vi "Script Name Wiring.vi"(6 "VI Name":string, 8 "error in":errorcluster, 9 "VI":refnum<vi>, 10 "Terminal Attributes":T1) -> (0 "error out":errorcluster)   [LabVIEW 2025, in "_Rescript.lvlib" / "Msg.lvlib" / "Msg.lvclass"]
uses:
  Msg.lvclass
  Terminal Attributes.ctl
  Attributes.ctl
  <vilib>/Utility/traverseref.llb/TRef TravTarget.ctl
  _Rescript.lvlib
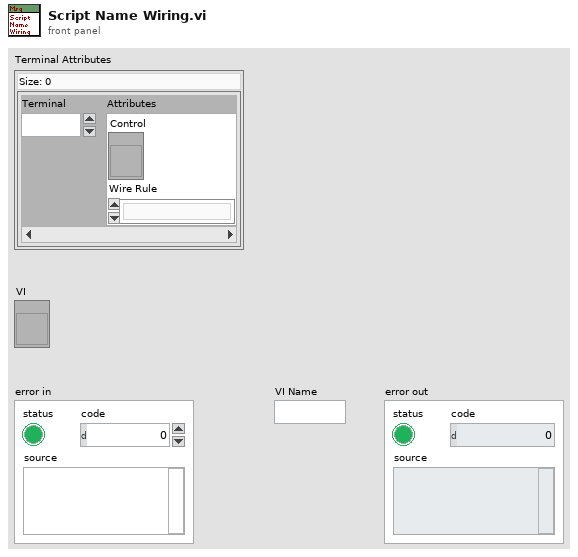
[diagram p1: front panel]
types:
  T1 = typedef "_Rescript.lvlib/Terminal Attributes.ctl" = map{i32, T2}
  T2 = typedef "_Rescript.lvlib/Attributes.ctl" = cluster{"Control":refnum<vi>, "Wire Rule":enum16{"Invalid Wire Rule", "Required", "Recommended", "Optional", "Dynamic Dispatch"}}
  T3 = typedef "TRef TravTarget.ctl" = enum16{"FP", "BD", "Other"}
  T4 = enum16{"Invalid Wire Rule", "Required", "Recommended", "Optional", "Dynamic Dispatch"}
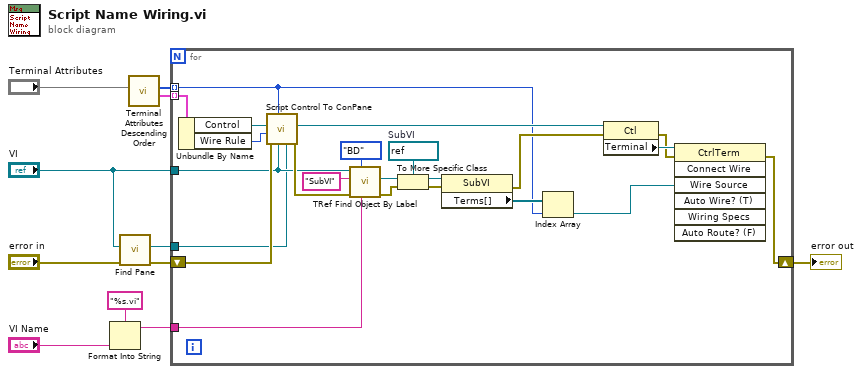
[diagram p0: block diagram]
diagram:
  n1 = Format Into String(format string="%s.vi", "VI Name") -> (resulting string=w4:string)  [unwired: 2 in, 1 out]
  n2 = call "Find Pane.vi"("error in"="error in", "VI Ref"="VI") -> ("error out"=w10:errorcluster, "Pane Ref"=w11:refnum<vi>)  [unwired: 8 in]
  n3 = call "Terminal Attributes Descending Order.vi"("Terminal Attributes"="Terminal Attributes") -> ("Attributes Descending Order"=w9:T2[], "Terminal Descending Order"=w8:i32[])  [unwired: 9 in]
  n4 = for {
    tunnel: w8 -> [w14] mode=indexing
    tunnel: w11 -> [w17]
    tunnel: "VI" -> [w18]
    shift-right: [w32] -> w7
    shift-left: w10 -> [w21]
    tunnel: w9 -> [w13] mode=indexing
    tunnel: w4 -> [w12]
    w30 = refnum<vi> refnum  # SubVI
    n5 = Unbundle By Name(w13) -> ("Control"=w16:refnum<vi>, "Wire Rule"=w15:T4)
    n6 = call "Script Control To ConPane.vi"("Pane"=w17, "VI"=w18, "Terminal"=w14, "error in"=w21, "Wire Rule"=w15, "Control To Duplicate"=w16) -> ("error out"=w20:errorcluster, "Duplicated Control"=w19:refnum<vi>)  [unwired: 4 in]
    n7 = call <vilib>:"TRef Find Object By Label.vi"("Label"=w12, "Traverse Target"=TRef_TravTarget."BD", "error in (no error)"=w20, "Class Name"="SubVI", "VI Ref"=w18) -> ("error out"=w29:errorcluster, "Found Obj Ref"=w24:refnum<vi>)  [unwired: 3 in, 2 out]
    n8 = To More Specific Class(target class=w30, reference=w24, error in=w29) -> (specific class reference=w27:refnum<vi>, error out=w26:errorcluster)
    n9 = property class="SubVI"(reference=w27, error in=w26) -> (error out=w22:errorcluster, "Terms[]"=w25:refnum<vi>[])  [unwired: 1 out]
    n10 = Index Array(array=w25, index=w14) -> (element=w23:refnum<vi>)
    n11 = property class="Ctl"(reference=w19, error in=w22) -> (error out=w33:errorcluster, "Terminal"=w34:refnum<vi>)  [unwired: 1 out]
    n12 = invoke class="CtrlTerm" method="Connect Wire"(reference=w34, error in=w33, "Wire Source"=w23) -> (error out=w32:errorcluster)  [unwired: 4 in, 6 out]
  }
  "error out" <- w7
